vi "DAQWriteData.vi"() -> ()   [LabVIEW 2017]
uses:
  <vilib>/DAQmx/write.llb/DAQmx Write (Analog 2D DBL NChan NSamp).vi
  <vilib>/DAQmx/create/channels.llb/DAQmx Create Channel (AO-Voltage-Basic).vi
  <vilib>/DAQmx/configure/timing.llb/DAQmx Timing (Sample Clock).vi
  <vilib>/DAQmx/miscellaneous.llb/DAQmx Fill In Error Info.vi
panel:
  in  "first data channel (1-based)":i32=1
  in  "Ref offline?":bool=TRUE
  in  "AO channels":tag="pciDAQ/ao0:2"
  in  "file paths":path[](array[path])
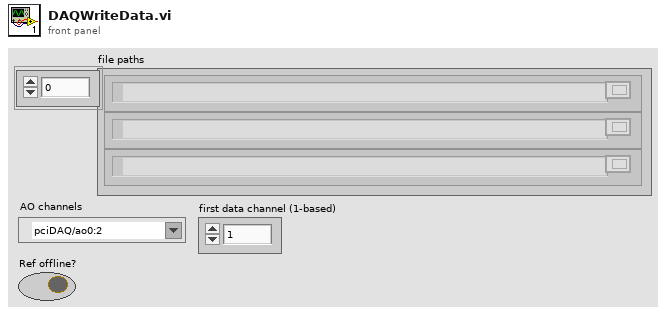
[diagram p1: front panel]
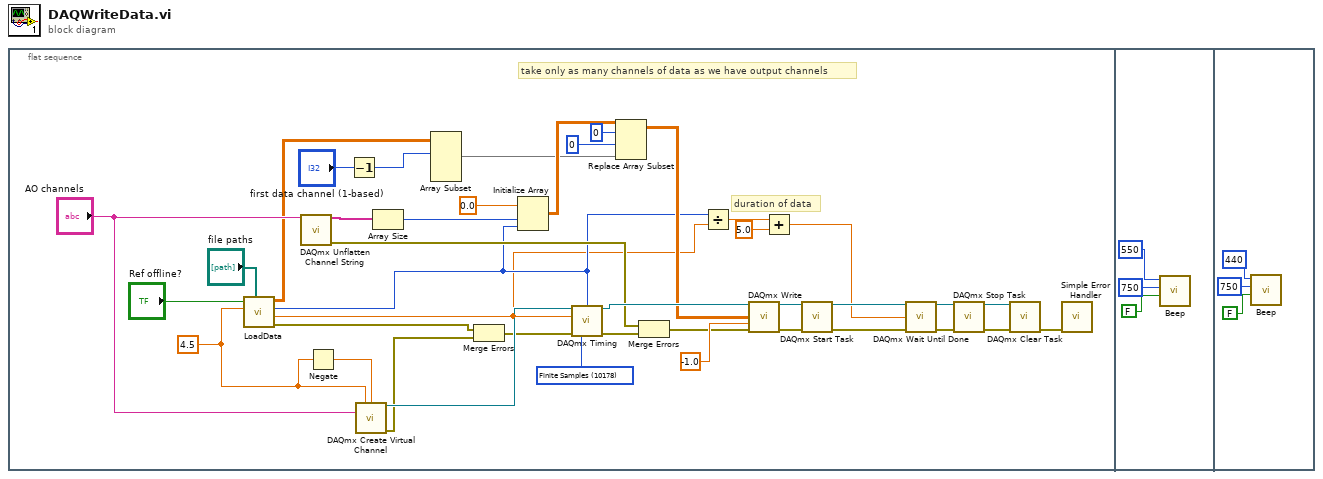
[diagram p0: block diagram]
diagram:
  n1 = flat-sequence {
    frame #0 {
      w38 = 10178 items=["Finite Samples"=10178, "Continuous Samples"=10123, "Hardware Timed Single Point"=12522] ("sample mode")
      w40 = 4.5
      # "duration of data"
      # "take only as many channels of data as we have output channels"
      n2 = call "LoadData.vi"("data files"="file paths", "max amplitude of\noutput"=w40, "CAR?"="Ref offline?") -> ("error out"=w18:errorcluster, "fs"=w9:dbl, "# samples"=w10:i32, "data"=w30:dbl[][])  [unwired: 3 in]
      n3 = call <vilib>:"DAQmx Unflatten Channel String.vi"("names in"="AO channels") -> ("names out"=w31:string[], "error out"=w15:errorcluster)  [unwired: 13 in]
      n4 = Negate(x=w40) -> (-x=w39:dbl)
      n5 = Decrement(x="first data channel (1-based)") -> (x-1=w29:i32)
      n6 = call-poly <vilib>:"DAQmx Create Virtual Channel.vi"("maximum value"=w40, "minimum value"=w39, "physical channels"="AO channels") -> ("task out"=w33:refnum<k21>, "error out"=w17:errorcluster)  [unwired: 11 in]
      n7 = Array Size(array=w31) -> (size(s)=w27:i32)
      n8 = Array Subset(array=w30, index (row)=w29) -> (w24:dbl[][])  [unwired: 3 in]
      n9 = Merge Errors(w18, w17) -> (w19:errorcluster)
      n10 = Initialize Array(0.0 ("element"), w27, w10) -> (w25:dbl[][])
      n11 = call-poly <vilib>:"DAQmx Timing.vi"("task/channels in"=w33, "sample mode"=w38, "samples per channel"=w10, "rate"=w9, "error in"=w19) -> ("task out"=w37:refnum<k21>, "error out"=w36:errorcluster)  [unwired: 9 in]
      n12 = Replace Array Subset(array=w25, new element=w24, index (row)=0, index (col)=0 ("disabled index (col)")) -> (w23:dbl[][])
      n13 = Merge Errors(w15, w36) -> (w16:errorcluster)
      n14 = Divide(x=w10, y=w9) -> (x/y=w8:dbl)
      n15 = call-poly <vilib>:"DAQmx Write.vi"("task/channels in"=w37, "data"=w23, "timeout"=-1.0, "error in"=w16) -> ("task out"=w14:refnum<k21>, "error out"=w13:errorcluster)  [unwired: 9 in, 1 out]
      n16 = Add(x=w8, y=5.0) -> (x+y=w6:dbl)
      n17 = call <vilib>:"DAQmx Start Task.vi"("task/channels in"=w14, "error in"=w13) -> ("task out"=w12:refnum<k21>, "error out"=w11:errorcluster)  [unwired: 12 in]
      n18 = call <vilib>:"DAQmx Wait Until Done.vi"("task/channels in"=w12, "timeout (sec)"=w6, "error in"=w11) -> ("task out"=w2:refnum<k21>, "error out"=w3:errorcluster)  [unwired: 11 in]
      n19 = call <vilib>:"DAQmx Stop Task.vi"("task/channels in"=w2, "error in"=w3) -> ("task out"=w5:refnum<k21>, "error out"=w4:errorcluster)  [unwired: 12 in]
      n20 = call <vilib>:"DAQmx Clear Task.vi"("task in"=w5, "error in"=w4) -> ("error out"=w1:errorcluster)  [unwired: 13 in]
      n21 = call <vilib>:"Simple Error Handler.vi"("error in (no error)"=w1) -> ()  [unwired: 4 in, 5 out]
    }
    frame #1 {
      n22 = call <vilib>:"Beep.vi"("use system alert? (T)"=FALSE, "duration (msec)"=u32 750, "frequency (Hz)"=u32 550) -> ()  [unwired: 9 in]
    }
    frame #2 {
      n23 = call <vilib>:"Beep.vi"("use system alert? (T)"=FALSE, "duration (msec)"=u32 750, "frequency (Hz)"=u32 440) -> ()  [unwired: 9 in]
    }
  }
